vi "RSZVB Set Pulse Time Stop.vi"(8 "error in (no error)":errorcluster {"code" format="%.0x"}, 9 "Time Stop (100.0e-6 seconds)":dbl=0.0001 format="%^.3e", 10 "Channel (1)":i32=1, 11 "VISA session":refnum<visa-resource-name>) -> (0 "error out":errorcluster {"code" format="%.0x"}, 3 "dup VISA session":refnum<visa-resource-name>)   [LabVIEW 2011]
doc: "This VI sets the stop time of the displayed time range relative to the trigger time.\n\nRemote-control command(s):\n[SENSe<Ch>:]PULSe:TIME:STOP <stop>"
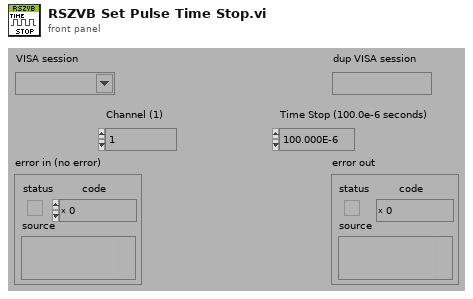
[diagram p1: front panel]
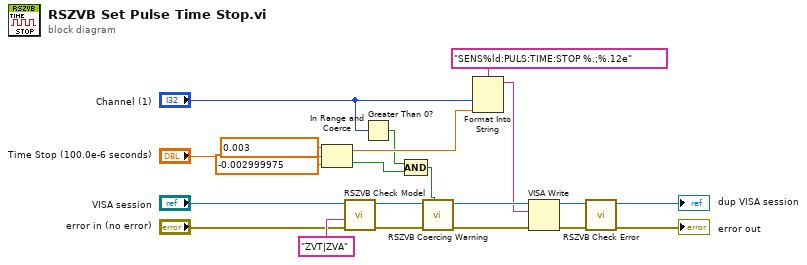
[diagram p0: block diagram]
diagram:
  n1 = In Range and Coerce(upper limit=0.003, x="Time Stop (100.0e-6 seconds)", lower limit=-0.002999975) -> (coerced(x)=w11:dbl, In Range?=w12:bool)
  n2 = call "RSZVB Check Model.vi"("error in (no error)"="error in (no error)", "Model"="ZVT|ZVA" ("Options"), "VISA session"="VISA session") -> ("error out"=w15:errorcluster, "dup VISA session"=w14:refnum<visa-resource-name>)  [unwired: 7 in]
  n3 = Greater Than 0?(x="Channel (1)") -> (x > 0?=w10:bool)
  n4 = Compound Arithmetic op=AND(w10, w12) -> (w9:bool)
  n5 = call "RSZVB Coercing Warning.vi"("In Range?"=w9, "error in (no error)"=w15, "VISA session"=w14) -> ("error out"=w19:errorcluster, "dup VISA session"=w20:refnum<visa-resource-name>)  [unwired: 7 in]
  n6 = Format Into String(format string="SENS%ld:PULS:TIME:STOP %.;%.12e", "Channel (1)", w11) -> (resulting string=w16:string)  [unwired: 2 in, 1 out]
  n7 = VISA Write(VISA resource name=w20, write buffer=w16, error in (no error)=w19) -> (VISA resource name out=w17:refnum<visa-resource-name>, error out=w18:errorcluster)  [unwired: 1 out]
  n8 = call "RSZVB Check Error.vi"("error in (no error)"=w18, "VISA session"=w17) -> ("error out"=→"error out":errorcluster, "dup VISA session"=→"dup VISA session":refnum<visa-resource-name>)  [unwired: 8 in]
